vi "espectro_hz_log_norm.vi"(9 "N FFT dBV":i32, 11 "X":dbl[](array[numeric])) -> (3 "FFT dB":cdb[](array[numeric]))   [LabVIEW 2020]
uses:
  <vilib>/Analysis/2dsp.llb/Real FFT.vi
  <vilib>/Analysis/NI_AALPro.lvlib
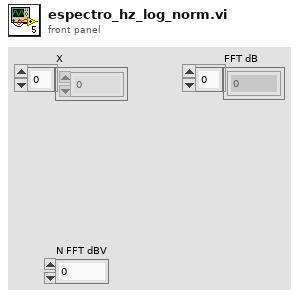
[diagram p1: front panel]
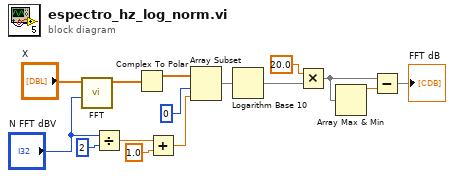
[diagram p0: block diagram]
diagram:
  n1 = call-poly <vilib>:"FFT.vi"("FFT size"="N FFT dBV", "X"="X") -> ("FFT {X}"=w8:cdb[])  [unwired: 8 in, 1 out]
  n2 = Divide(x="N FFT dBV", y=2) -> (x/y=w11:dbl)
  n3 = Complex To Polar(r * e^(i*theta)=w8) -> (r=w7:dbl[])  [unwired: 1 out]
  n4 = Add(x=w11, y=1.0) -> (x+y=w9:dbl)
  n5 = Array Subset(array=w7, index=0, length=w9) -> (w4:dbl[])
  n6 = Logarithm Base 10(1:w4) -> (0:w15:dbl[])
  n7 = Multiply(x=20.0, y=w15) -> (x*y=w3:dbl[])
  n8 = Array Max & Min(array=w3) -> (max value=w2:dbl)  [unwired: 3 out]
  n9 = Subtract(x=w3, y=w2) -> (x-y=→"FFT dB":dbl[])
